vi "Create.vi"(4 "Id (-1 = undefined)":i32=-1, 5 "Test Suite in":refnum<class "Test Suite.lvclass">, 6 "Package (\"\" = undefined)":string, 8 "error in (no error)":errorcluster, 11 "Name":string) -> (0 "error out":errorcluster, 3 "Test Suite":refnum<class "Test Suite.lvclass">)   [LabVIEW 2013, in "JUnit XML.lvlib" / "Test Suite.lvclass"]
doc: "Creates a new instance of the <B>Test Suite</B> class."
uses:
  Test Suite.lvclass
  Test Suite.lvclass/Test Suite.ctl
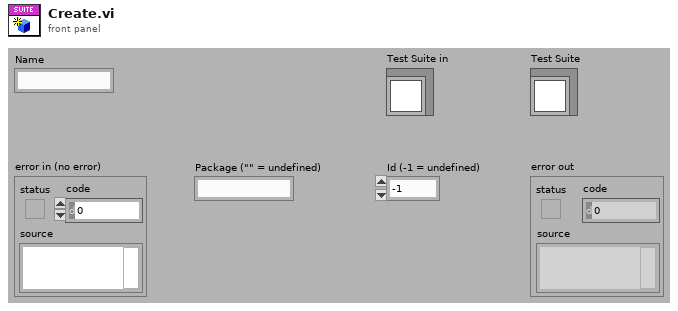
[diagram p1: front panel]
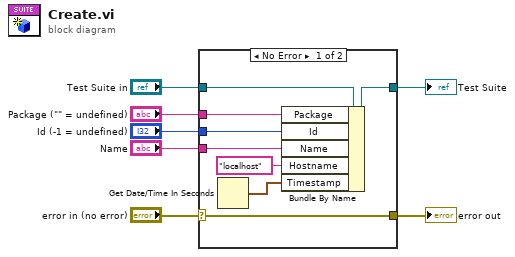
[diagram p0: block diagram]
diagram:
  n1 = case shown="No Error" "error in (no error)" {
    selector: "error in (no error)" -> [w15 w17]
    tunnel: [w15 w17] -> w6
    tunnel: [w13 w16] -> w4
    tunnel: "Test Suite in" -> [w14 w16]
    tunnel: "Package (\"\" = undefined)" -> [w12 _]
    tunnel: "Id (-1 = undefined)" -> [w11 _]
    tunnel: "Name" -> [w10 _]
    frame No Error {
      n2 = Get Date/Time In Seconds() -> (seconds since 1Jan1904=w9:timestamp)
      n3 = Bundle By Name(cluster=w14, "Package"=w12, "Id"=w11, "Name"=w10, "Hostname"="localhost", "Timestamp"=w9) -> (w13:refnum<class "Test Suite.lvclass">)
    }
    frame Error {
    }
  }
  "error out" <- w6
  "Test Suite" <- w4
